vi "Main.vi"() -> ()   [LabVIEW 2021]
panel:
  in  "stop":bool
  out "Indicator":bool
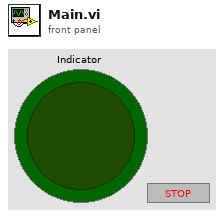
[diagram p1: front panel]
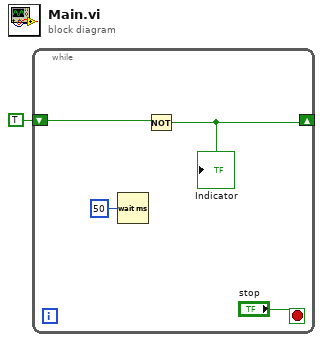
[diagram p0: block diagram]
diagram:
  n1 = while {
    shift-right: [w4] -> _
    shift-left: TRUE -> [w5]
    stop <- "stop" stop-if-true
    n2 = Wait (ms)(milliseconds to wait=u32 50) -> ()  [unwired: 1 out]
    n3 = Not(x=w5) -> (.not. x?=w4:bool)
    "Indicator" <- w4
  }
